vi "PH_Beckhoff_PP_Control.declare Tags.vi"() -> (0 "Data in cluster":T1={"Default Values"={"Sonderklemmen Inputs"=[], "Analog Inputs"=[], "Analog Outputs"=[], "Digital Inputs"=[], "Digital Outputs"=[]}, "Description"="", "Hardware configured?"=TRUE, "Activate Change Manager?"=FALSE, "Difference to handle an analog input as change"=1})   [LabVIEW 2014, in "PH_Beckhoff_PP_Control.lvlib"]
doc: "This VI declares the tagnames and sets the scaling of the tags of this class."
uses:
  PH_Beckhoff_PP_Control.lvlib
  PH_Beckhoff/PH_Beckhoff.constructor Data in.ctl
  PH_Beckhoff/PH_Beckhoff.Values.ctl
  PH_Beckhoff/PH_Beckhoff.Sonderklemmen Inputs.ctl
  PH_Beckhoff/PH_Beckhoff.Analog Inputs.ctl
  PH_Beckhoff/PH_Beckhoff.Scaling Type.ctl
  PH_Beckhoff/PH_Beckhoff.Analog Outputs.ctl
  PH_Beckhoff/PH_Beckhoff.Digital Inputs.ctl
  PH_Beckhoff/PH_Beckhoff.Digital Outputs.ctl
  PH_Beckhoff/PH_Beckhoff.lvlib
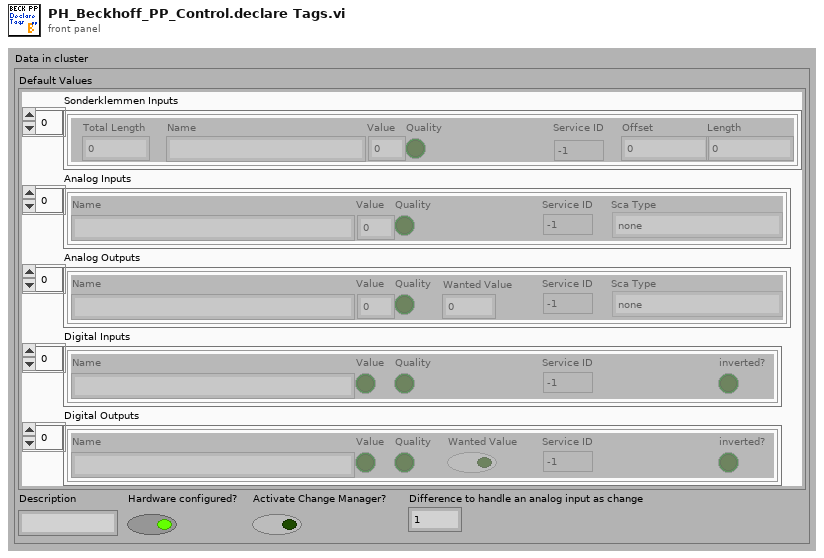
[diagram p1: front panel]
types:
  T1 = typedef "PH_Beckhoff.lvlib/PH_Beckhoff.constructor Data in.ctl" = cluster{"Default Values":T2, "Description":string, "Hardware configured?":bool, "Activate Change Manager?":bool, "Difference to handle an analog input as change":u32}
  T2 = typedef "PH_Beckhoff.lvlib/PH_Beckhoff.Values.ctl" = cluster{"Sonderklemmen Inputs":T3, "Analog Inputs":T4, "Analog Outputs":T6, "Digital Inputs":T7, "Digital Outputs":T8}
  T3 = typedef "PH_Beckhoff.lvlib/PH_Beckhoff.Sonderklemmen Inputs.ctl" = cluster{"Total Length":u32, "Name":string, "Value":u64, "Quality":bool, "Service ID":i32, "Offset":u32, "Length":u32}[]
  T4 = typedef "PH_Beckhoff.lvlib/PH_Beckhoff.Analog Inputs.ctl" = cluster{"Name":string, "Value":u32, "Quality":bool, "Service ID":i32, "Sca Type":T5}[]
  T5 = typedef "PH_Beckhoff.lvlib/PH_Beckhoff.Scaling Type.ctl" = enum16{"none", "0 ... 15 Bit -> 0 ... 5", "0 ... 15 Bit -> 0 ... 10", "0 ... 15 Bit -> 0 ... 25", "0 ... 15 Bit -> 4 ... 20", "0 ... 15 Bit -> 0 ... 1", "0 ... 15 Bit -> 0 ... 20000", "0 ... 15 Bit -> 0 ... 24000"}
  T6 = typedef "PH_Beckhoff.lvlib/PH_Beckhoff.Analog Outputs.ctl" = cluster{"Name":string, "Value":u32, "Quality":bool, "Wanted Value":u32, "Service ID":i32, "Sca Type":T5}[]
  T7 = typedef "PH_Beckhoff.lvlib/PH_Beckhoff.Digital Inputs.ctl" = cluster{"Name":string, "Value":bool, "Quality":bool, "Service ID":i32, "inverted?":bool}[]
  T8 = typedef "PH_Beckhoff.lvlib/PH_Beckhoff.Digital Outputs.ctl" = cluster{"Name":string, "Value":bool, "Quality":bool, "Wanted Value":bool, "Service ID":i32, "inverted?":bool}[]
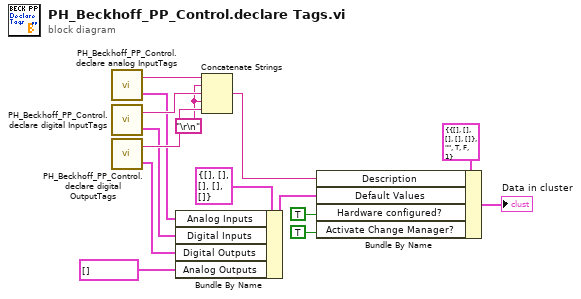
[diagram p0: block diagram]
diagram:
  w7 = "\r\n"
  n1 = call "PH_Beckhoff_PP_Control.declare analog InputTags.vi"() -> ("Analog Inputs"=w3:T4, "Description"=w6:string)
  n2 = call "PH_Beckhoff_PP_Control.declare digital InputTags.vi"() -> ("Digital Inputs"=w4:T7, "Description"=w10:string)
  n3 = call "PH_Beckhoff_PP_Control.declare digital OutputTags.vi"() -> ("Digital Outputs"=w5:T8, "Description"=w9:string)
  n4 = Bundle By Name(cluster=T2 {"Sonderklemmen Inputs"=[], "Analog Inputs"=[], "Analog Outputs"=[], "Digital Inputs"=[], "Digital Outputs"=[]} ("Dummy Default Values"), "Analog Inputs"=w3, "Digital Inputs"=w4, "Digital Outputs"=w5, "Analog Outputs"=T6 []) -> (w12:T2)
  n5 = Concatenate Strings(w6, w7, w10, w7, w9) -> (w8:string)
  n6 = Bundle By Name(cluster=T1 {"Default Values"={"Sonderklemmen Inputs"=[], "Analog Inputs"=[], "Analog Outputs"=[], "Digital Inputs"=[], "Digital Outputs"=[]}, "Description"="", "Hardware configured?"=TRUE, "Activate Change Manager?"=FALSE, "Difference to handle an analog input as change"=1} ("Dummy data in cluster"), "Description"=w8, "Default Values"=w12, "Hardware configured?"=TRUE, "Activate Change Manager?"=TRUE) -> (→"Data in cluster":T1)
